vi "CoordRunCaliper.vi"(8 "error in (no error)":errorcluster, 10 "CoordinatteEntry In":T1={"ProcessSetting"=[], "Project Name"="Parttern", "AnalysisSetting"=[], "Coord?"=FALSE, "OriginPointInfo"={"Output Original"=FALSE, "Origin Name"="", "Angle"=0.0, "Mode"=0, "OriginPoint"={"X"=0.0, "Y"=0.0}}, "CaliperSetting"=[], "CoordIndex"=[]} {"CaliperSetting"."CaliperEntry"."CaliperType" items=["Distance", "Mid Point", "Perpendicular Projection", "Lines Intersection", "Angle from Horizontal", "Angle from Vertical", "Angle Defined by 3 Points", "Angle Defined by 4 Points", "Bissecting Line", "Mid Line", "Center of Mass", "Area", "Line Fit", "Circle Fit", "Ellipse Fit"]; "OriginPointInfo"."Mode" items=["Horizontal Motion", "Vertical Motion", "Horizontal and Vertical Motion", "Horizontal. Vertical and Angular Motion"]; "AnalysisSetting"."ROI"."Contours"."Type" items=["No Selection", "Point", "Line", "Rectangle", "Oval", "Polygon", "Freehand Region", "Annulus", "Unused2", "Unused3", "Broken Line", "Freehand Line", "Rotated Rectangle"]}) -> (0 "error out":errorcluster, 2 "CoordinatteEntry Out":T1={"ProcessSetting"=[], "Project Name"="Parttern", "AnalysisSetting"=[], "Coord?"=FALSE, "OriginPointInfo"={"Output Original"=FALSE, "Origin Name"="", "Angle"=0.0, "Mode"=0, "OriginPoint"={"X"=0.0, "Y"=0.0}}, "CaliperSetting"=[], "CoordIndex"=[]} {"CaliperSetting"."CaliperEntry"."CaliperType" items=["Distance", "Mid Point", "Perpendicular Projection", "Lines Intersection", "Angle from Horizontal", "Angle from Vertical", "Angle Defined by 3 Points", "Angle Defined by 4 Points", "Bissecting Line", "Mid Line", "Center of Mass", "Area", "Line Fit", "Circle Fit", "Ellipse Fit"]; "OriginPointInfo"."Mode" items=["Horizontal Motion", "Vertical Motion", "Horizontal and Vertical Motion", "Horizontal. Vertical and Angular Motion"]; "AnalysisSetting"."ROI"."Contours"."Type" items=["No Selection", "Point", "Line", "Rectangle", "Oval", "Polygon", "Freehand Region", "Annulus", "Unused2", "Unused3", "Broken Line", "Freehand Line", "Rotated Rectangle"]})   [LabVIEW 2019]
uses:
  Control/CoordinatteEntry.ctl
  Process/Controls/Process_Setting.ctl
  Ctrl/VisionProcessName.ctl
  Control/CoordinateAnalysisSetting.ctl
  Control/CoordinateCaliperSetting.ctl
  Caliper/Controls/CaliperDataEntry.ctl
  Caliper/Controls/CaliperType.ctl
  Caliper/Controls/SelectionListEntry.ctl
  Caliper/Controls/SelectionListEntryPointType.ctl
  Caliper/Controls/CaliperResult.ctl
  Caliper/Controls/Caliper_Entry_FGV_Action.ctl
  Caliper/Controls/AnalysisResultPointsAction.ctl
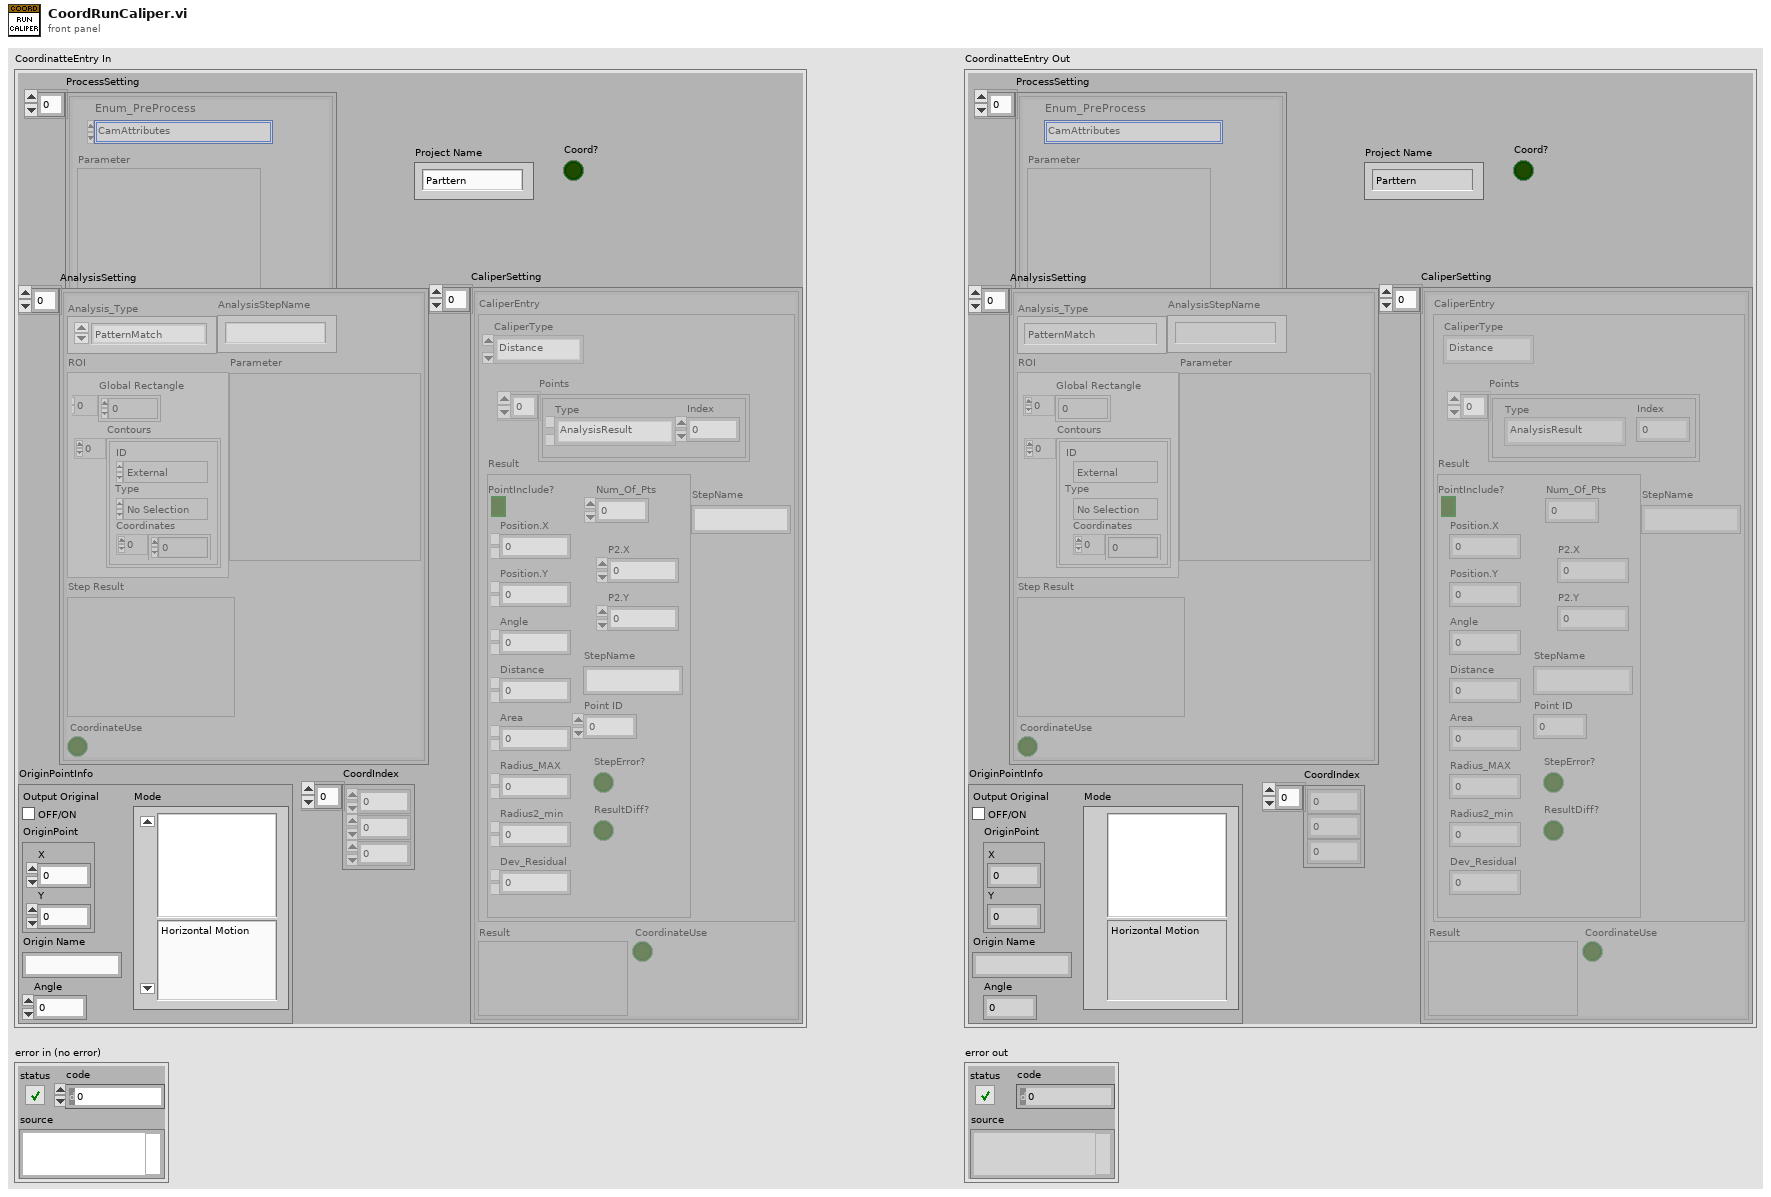
[diagram p1: front panel]
types:
  T1 = typedef "CoordinatteEntry.ctl" = cluster{"ProcessSetting":T2[], "Project Name":string, "AnalysisSetting":T4[], "Coord?":bool, "OriginPointInfo":cluster{"Output Original":bool, "Origin Name":string, "Angle":dbl, "Mode":u16, "OriginPoint":cluster{"X":dbl, "Y":dbl}}, "CaliperSetting":T6[], "CoordIndex":i32[]}
  T2 = typedef "Process_Setting.ctl" = cluster{"Enum_PreProcess":T3, "Parameter":string}
  T3 = typedef "VisionProcessName.ctl" = enum16{"*CamParameter*", "CamAttributes", "*Preprocess*", "CG_Brightness", "C_Plane Extraction", "C_Threshold", "G_Lookup Table", "G_Threshold"}
  T4 = typedef "CoordinateAnalysisSetting.ctl" = cluster{"Analysis_Type":enum16{"PatternMatch", "Straight Edge"}, "ROI ":T5, "Parameter":variant, "Step Result":variant, "AnalysisStepName":string, "CoordinateUse":bool}
  T5 = typedef "ROI Descriptor" = cluster{"Global Rectangle":i32[], "Contours":cluster{"ID":enum32{"External", "Internal"}, "Type":u32, "Coordinates":i32[]}[]}
  T6 = typedef "CoordinateCaliperSetting.ctl" = cluster{"Result":variant, "CoordinateUse":bool, "CaliperEntry":T7}
  T7 = typedef "CaliperDataEntry.ctl" = cluster{"CaliperType":T8, "Points":T9[], "Result":T11, "StepName":string}
  T8 = typedef "CaliperType.ctl" = u32
  T9 = typedef "SelectionListEntry.ctl" = cluster{"Type":T10, "Index":i32}
  T10 = typedef "SelectionListEntryPointType.ctl" = enum16{"AnalysisResult", "CaliperResult"}
  T11 = typedef "CaliperResult.ctl" = cluster{"PointInclude?":bool, "Num_Of_Pts":u8, "Position.X":dbl, "Position.Y":dbl, "Angle":dbl, "Distance":dbl, "Area":dbl, "Radius_MAX":dbl, "Radius2_min":dbl, "Dev_Residual":dbl, "P2.X":dbl, "P2.Y":dbl, "StepName":string, "Point ID":u8, "StepError?":bool, "ResultDiff?":bool}
  T12 = typedef "AnalysisResultPointsAction.ctl" = enum16{"Init", "Add", "Delete", "ReplaceAll", "ReadAll", "Close"}
  T13 = typedef "Caliper_Entry_FGV_Action.ctl" = enum16{"Init", "Close", "Add", "Delete", "ReplaceAll", "ReadAll"}
  T14 = typedef "Analysis_Result_To_Caliper.ctl" = cluster{"PointName":string, "Position_X":dbl, "Position_Y":dbl}
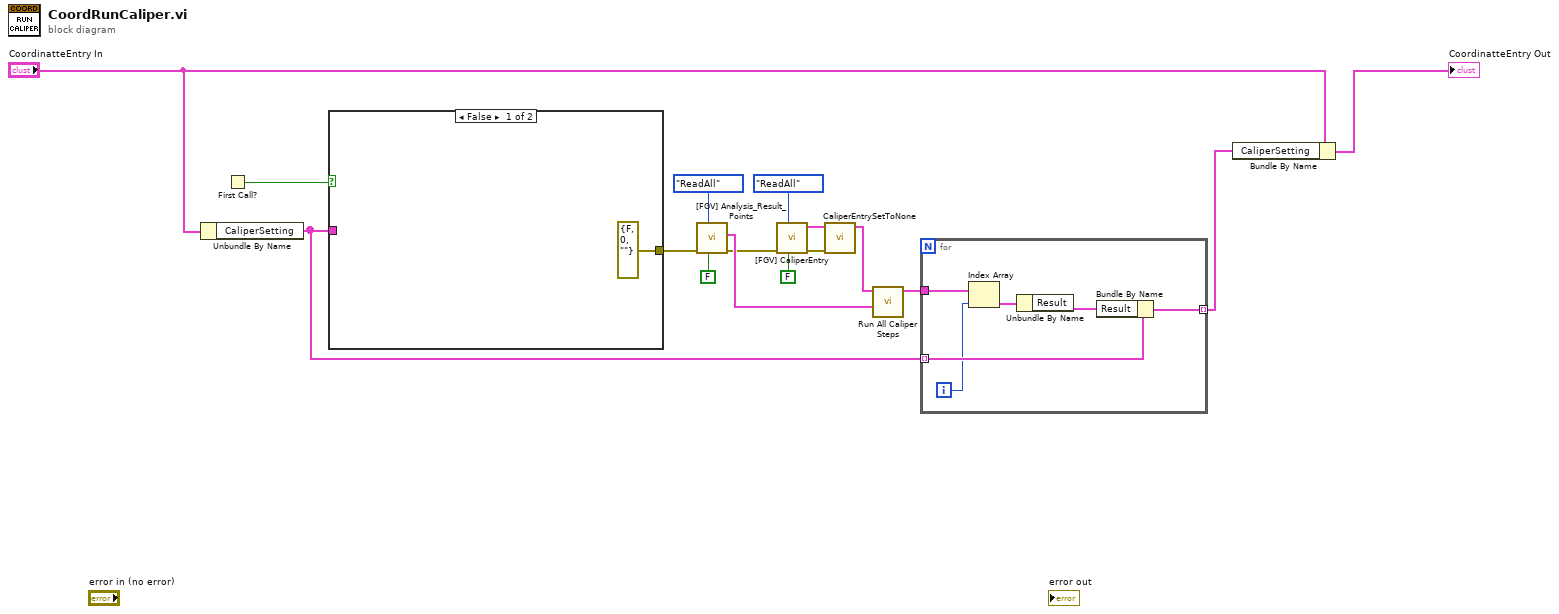
[diagram p0: block diagram]
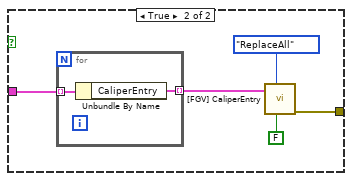
[diagram p2: hidden frame]
diagram:
  n1 = Unbundle By Name("CoordinatteEntry In") -> ("CaliperSetting"=w1:T6[])
  n2 = First Call?() -> (First Call?: T/F=w5:bool)
  n3 = case shown="False" w5 {
    tunnel: [errorcluster {"status"=FALSE, "code"=0, "source"=""} ("error out") w20] -> w4
    tunnel: w1 -> [_ w19]
    frame False {
    }
    frame True {
      n4 = for {
        tunnel: w19 -> [w24] mode=indexing
        tunnel: [w23] -> w18 mode=indexing
        n5 = Unbundle By Name(w24) -> ("CaliperEntry"=w23:T7)
      }
      n6 = call "[FGV] CaliperEntry.vi"("CoordSystemRun"=FALSE, "Action"=Caliper_Entry_FGV_Action."ReplaceAll", "CaliperEntriesIn"=w18) -> ("error out"=w20:errorcluster)  [unwired: 7 in, 1 out]
    }
  }
  n7 = call "[FGV] Analysis_Result_Points.vi"("CoordSystemRun"=FALSE, "Action"=AnalysisResultPointsAction."ReadAll", "error in (no error)"=w4) -> ("error out"=w3:errorcluster, "Analysis_Point_Result Out"=w14:T14[])  [unwired: 7 in]
  n8 = call "[FGV] CaliperEntry.vi"("CoordSystemRun"=FALSE, "Action"=Caliper_Entry_FGV_Action."ReadAll", "error in (no error)"=w3) -> ("error out"=w2:errorcluster, "AllCaliperEntries"=w10:T7[])  [unwired: 7 in]
  n9 = call "CaliperEntrySetToNone.vi"("error in (no error)"=w2, "CaliperEntryList"=w10) -> ("CaliperEntryOut"=w8:T7[])  [unwired: 8 in, 1 out]
  n10 = call "Run All Caliper Steps.vi"("Analysis_Point_Result"=w14, "CaliperEntryList"=w8) -> ("CaliperEntryOut"=w7:T7[])  [unwired: 9 in]
  n11 = for {
    tunnel: w1 -> [w30] mode=indexing
    tunnel: w7 -> [w29]
    tunnel: [w26] -> w6 mode=indexing
    i -> [w25]
    n12 = Index Array(array=w29, index=w25) -> (element=w28:T7)
    n13 = Unbundle By Name(w28) -> ("Result"=w27:T11)
    n14 = Bundle By Name(cluster=w30, "Result"=w27) -> (w26:T6)
  }
  n15 = Bundle By Name(cluster="CoordinatteEntry In", "CaliperSetting"=w6) -> (→"CoordinatteEntry Out":T1)
